vi "HumanNetwork.vi"(8 "error in (no error)":errorcluster) -> (0 "error out":errorcluster)   [LabVIEW 2023]
doc: "Human Network\n\nInput\n --Error in \n\nOutput\n --Error out"
uses:
  HumanGlobal.vi
  <vilib>/Rock Robotics/Network Tables/NT Read Number.vi
  <vilib>/Rock Robotics/Network Tables/NT Read Boolean.vi
  <vilib>/Rock Robotics/Network Tables/NT Write String.vi
  <vilib>/Rock Robotics/Network Tables/NT Write Boolean.vi
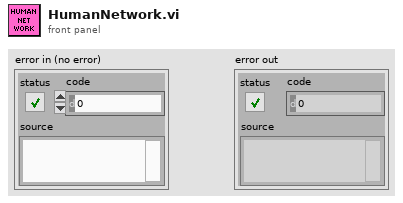
[diagram p1: front panel]
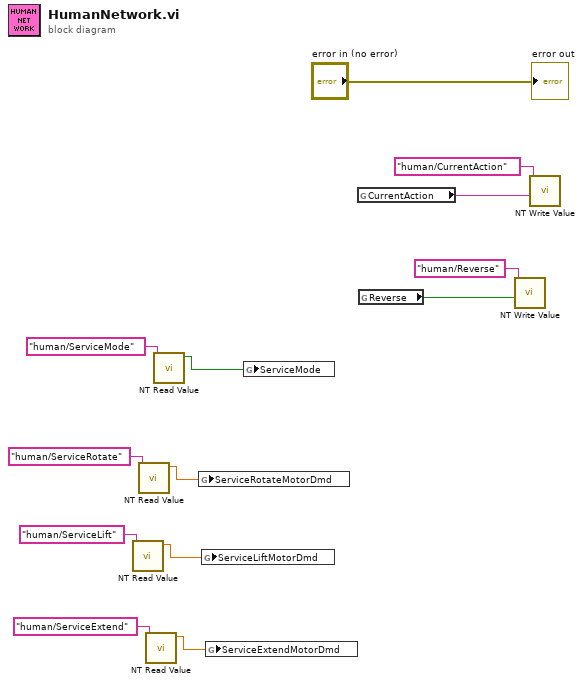
[diagram p0: block diagram]
diagram:
  n1 = call-poly <vilib>:"NT Read Value.vi"("name"="human/ServiceLift") -> ("value"=w4:dbl)  [unwired: 8 in, 2 out]
  n2 = call-poly <vilib>:"NT Read Value.vi"("name"="human/ServiceRotate") -> ("value"=w6:dbl)  [unwired: 8 in, 2 out]
  n3 = call-poly <vilib>:"NT Read Value.vi"("name"="human/ServiceExtend") -> ("value"=w2:dbl)  [unwired: 8 in, 2 out]
  n4 = call-poly <vilib>:"NT Read Value.vi"("name"="human/ServiceMode") -> ("value"=w7:bool)  [unwired: 8 in, 2 out]
  n5 = global write "HumanGlobal.vi" "ServiceRotateMotorDmd"(w6) -> ()
  n6 = global write "HumanGlobal.vi" "ServiceLiftMotorDmd"(w4) -> ()
  n7 = global write "HumanGlobal.vi" "ServiceExtendMotorDmd"(w2) -> ()
  n8 = global write "HumanGlobal.vi" "ServiceMode"(w7) -> ()
  n9 = global read "HumanGlobal.vi" "CurrentAction"() -> (w10:string)
  n10 = global read "HumanGlobal.vi" "Reverse"() -> (w12:bool)
  n11 = call-poly <vilib>:"NT Write Value.vi"("value"=w12, "name"="human/Reverse") -> ()  [unwired: 9 in, 1 out]
  n12 = call-poly <vilib>:"NT Write Value.vi"("value"=w10, "name"="human/CurrentAction") -> ()  [unwired: 9 in, 1 out]
  "error out" <- "error in (no error)"
